vi "Get Channel Settings UI.vi"(8 "error in (no error)":errorcluster, 11 "Component UI in":refnum<class "Component User Interface.lvclass">) -> (0 "error out":errorcluster, 2 "Channel Settings UI":refnum<class "User Interface.lvclass">, 3 "Component UI out":refnum<class "Component User Interface.lvclass">)   [LabVIEW 2017, in "DSF Core.lvlib" / "Component User Interface.lvclass"]
uses:
  Component User Interface.lvclass
  User Interface/User Interface.lvclass
  Component User Interface.lvclass/Component User Interface.ctl
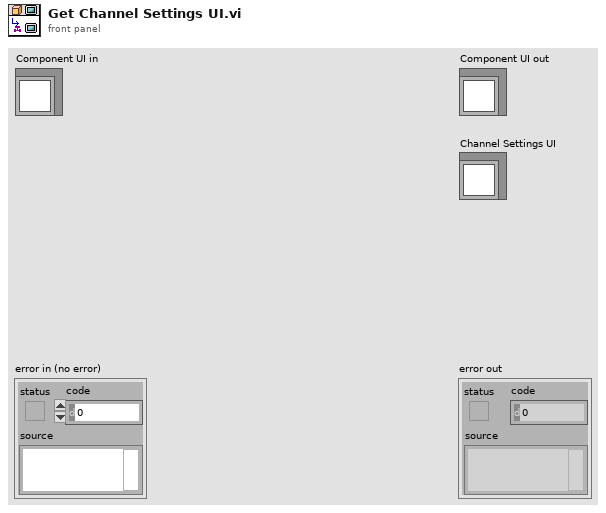
[diagram p1: front panel]
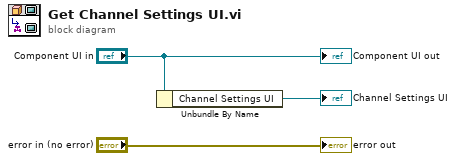
[diagram p0: block diagram]
diagram:
  n1 = Unbundle By Name("Component UI in") -> ("Channel Settings UI"=→"Channel Settings UI":refnum<class "User Interface.lvclass">)
  "error out" <- "error in (no error)"
  "Component UI out" <- "Component UI in"
